vi "GetTerms3.vi"(0 "XRef":T11, 1 "State In":T9) -> (14 "Terms":T1)   [LabVIEW 2012, in "CRefScripting.lvlib" / "CRef Label Node.xnode"]
doc: "This ability VI is used to describe your terminals to LabVIEW. Terms is an array of clusters describing the XNode's terminals.\n ID: A unique string identifying the terminal.\n Name: The name of the terminal visible to the user. Remember to localize it.\n Type: The data type of the terminal (as a Variant). The data put in the variant will be used as the default for the input terminal if it's left unwired.\n Bounds: A rectangle defining the bounds of the terminal relative to the bounds of the XNode. The bounds must be within the bounds of the XNode, and for whiskers to draw properly, they must be flush with at least one side of the XNode.\n Input?: Indicates whether or not this terminals is an input.\n Required?: Indicates whether the user must wire this terminal for the XNode to not be broken. Ignored on outputs.\n Recommended?: Indicates whether the terminal is recommended.\n Hidden?: Indicates whether the terminal is hidden. When a terminal is hidden, it cannot be wired to via user interaction or scripting. However, if it is already wired to when the hidden flag is changed to true, it will remain wired.\n Adaptive?: Indicates that the term should change to match the type of its source if it is wired.\n Direction?: Indicates what direction the wire stub should point. Choose auto to let LV decide based on the terms bounds being on the nodes edge.\n \n The IDs are used by LabVIEW to keep track of your terminals. When you respecify your terminals, LabVIEW can tell whther terminals are new, deleted, or moved by the unique IDs. The order is irrelevant. If you move a terminal, then any wire connected to it will move with it.\n \n If you want to update your terminals, you should return the UpdateTerms reply in one of your ability VIs.\n\nDefault behavior: None.\n\nThis ability does not provide UI and OS messages are not handled."
uses:
  CRef Label Node.xnode
  <vilib>/XNodeSupport/XNodeXNodeRef.ctl
  State.ctl
  Core/Master Types.ctl
  <vilib>/XNodeSupport/XNodeTerm3Array.ctl
  <vilib>/XNodeSupport/XNodeTerm3.ctl
  <vilib>/XNodeSupport/XNodeString.ctl
  <vilib>/XNodeSupport/XNodeVariant.ctl
  <vilib>/XNodeSupport/XNodeRect32.ctl
  <vilib>/XNodeSupport/XNodeInt.ctl
  <vilib>/XNodeSupport/XNodeBool.ctl
  <vilib>/XNodeSupport/XNodeTermDirection.ctl
  <vilib>/XNodeSupport/NI_XNodeSupport.lvlib
  CRef.lvlib
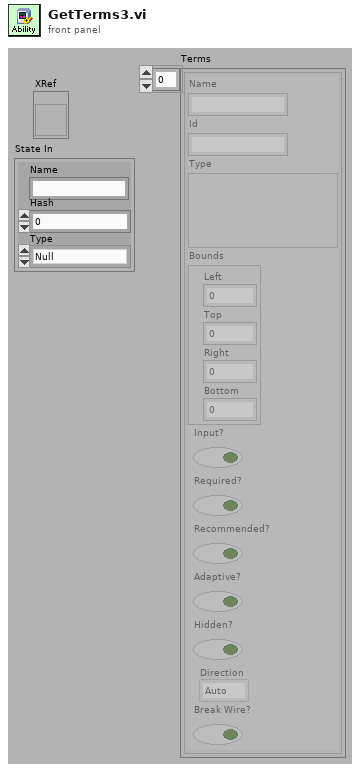
[diagram p1: front panel]
types:
  T1 = typedef "NI_XNodeSupport.lvlib/XNodeTerm3Array.ctl" = T2[]
  T2 = typedef "NI_XNodeSupport.lvlib/XNodeTerm3.ctl" = cluster{"Name":T3, "Id":T3, "Type":T4, "Bounds":T5, "Input?":T7, "Required?":T7, "Recommended?":T7, "Adaptive?":T7, "Hidden?":T7, "Direction":T8, "Break Wire?":T7}
  T3 = typedef "NI_XNodeSupport.lvlib/XNodeString.ctl" = string
  T4 = typedef "NI_XNodeSupport.lvlib/XNodeVariant.ctl" = variant
  T5 = typedef "NI_XNodeSupport.lvlib/XNodeRect32.ctl" = cluster{"Left":T6, "Top":T6, "Right":T6, "Bottom":T6}
  T6 = typedef "NI_XNodeSupport.lvlib/XNodeInt.ctl" = i32
  T7 = typedef "NI_XNodeSupport.lvlib/XNodeBool.ctl" = bool
  T8 = typedef "NI_XNodeSupport.lvlib/XNodeTermDirection.ctl" = enum32{"Auto", "Up", "Down", "Left", "Right", "Center"}
  T9 = typedef "CRefScripting.lvlib/CRef Label Node.xnode/State.ctl" = cluster{"Name":string, "Hash":u32, "Type":T10}
  T10 = typedef "CRef.lvlib/Master Types.ctl" = enum8{"Null", "Boolean", "U8", "I8", "U16", "I16", "U32", "I32", "U64", "I64", "Single", "Double", "Extended", "CSG", "CDB", "CXT", "Boolean(Def)", "U8(Def)", "I8(Def)", "U16(Def)", "I16(Def)", "U32(Def)", "I32(Def)", "Reserved Def", "Reserved Def1", "Single(Def)", "Double(Def)", "Reserved Def2", "Reserved Def3", "Reserved Def4", "Reserved Def5", "Unsigned(Def)", "Signed(Def)", "Real(Def)", "Reserved Def6", "Numeric(Def)", "String"}
  T11 = typedef "NI_XNodeSupport.lvlib/XNodeXNodeRef.ctl" = refnum<vi>
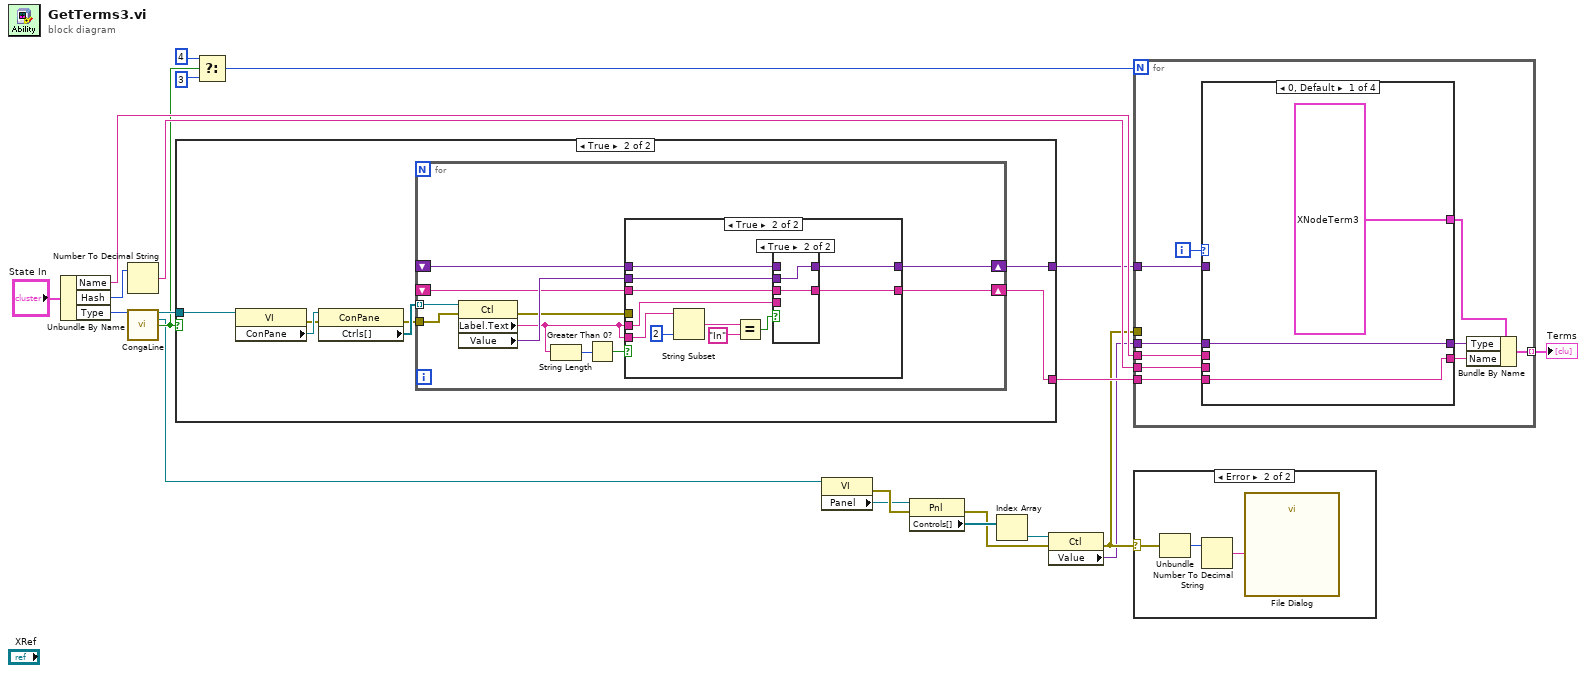
[diagram p0: block diagram]
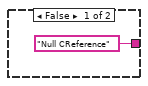
[diagram p3: hidden frame]
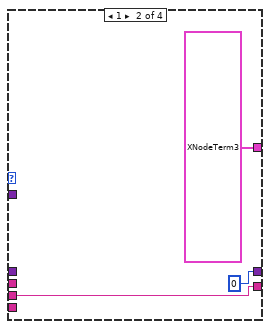
[diagram p6: hidden frame]
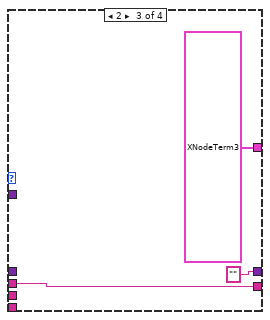
[diagram p7: hidden frame]
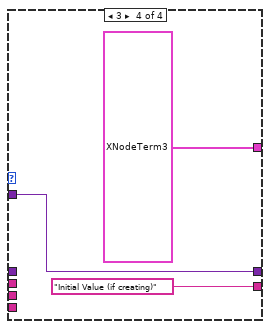
[diagram p8: hidden frame]
diagram:
  n1 = Unbundle By Name("State In") -> ("Name"=w18:string, "Hash"=w17:u32, "Type"=w20:T10)
  n2 = Number To Decimal String(number=w17) -> (decimal integer string=w16:string)  [unwired: 1 in]
  n3 = call "CongaLine.vi"("Type"=w20) -> ("vi reference"=w19:refnum<vi>, "CReference Ctl"=w8:refnum<vi>, "implemented?"=w9:bool)  [unwired: 11 in, 1 out]
  n4 = case shown="True" w9 {
    tunnel: w19 -> [_ w29]
    tunnel: [_ w26] -> w14
    tunnel: ["Null CReference" ("Label.ClassName") w25] -> w13
    frame False {
    }
    frame True {
      n5 = property class="VI"(reference=w29) -> (error out=w24:errorcluster, "ConPane"=w28:refnum<vi>)  [unwired: 1 in, 1 out]
      n6 = property class="ConPane"(reference=w28, error in=w24) -> (error out=w23:errorcluster, "Ctrls[]"=w27:refnum<vi>[])  [unwired: 1 out]
      n7 = for {
        tunnel: w27 -> [w40] mode=indexing
        shift-right: [w36] -> w26
        shift-left: _ -> [w35]
        shift-right: [w33] -> w25
        shift-left: _ -> [w32]
        tunnel: w23 -> [w31]
        n8 = property class="Ctl"(reference=w40, error in=w31) -> (error out=w30:errorcluster, "Label.Text"=w34:string, "Value"=w37:variant)  [unwired: 1 out]
        n9 = String Length(string=w34) -> (length=w39:i32)
        n10 = Greater Than 0?(x=w39) -> (x > 0?=w38:bool)
        n11 = case shown="True" w38 {
          tunnel: w37 -> [_ w48]
          tunnel: w34 -> [_ w52]
          tunnel: [w42 w47] -> w36
          tunnel: w35 -> [w42 w46]
          tunnel: w34 -> [_ w45]
          tunnel: [w41 w44] -> w33
          tunnel: w32 -> [w41 w43]
          tunnel: w30 -> [_ _]
          frame False {
          }
          frame True {
            n12 = String Subset(string=w52, length (rest)=2 ("length (rest)")) -> (substring=w51:string)  [unwired: 1 in]
            n13 = Equal?(x=w51, y="In") -> (x = y?=w49:bool)
            n14 = case shown="True" w49 {
              tunnel: w48 -> [_ w57]
              tunnel: [w55 w57] -> w47
              tunnel: w46 -> [w55 _]
              tunnel: [w54 w56] -> w44
              tunnel: w45 -> [w54 _]
              tunnel: w43 -> [_ w56]
              frame False {
              }
              frame True {
              }
            }
          }
        }
      }
    }
  }
  n15 = Select(t=4, s=w9, f=3) -> (s? t:f=w10:i32)
  n16 = property class="VI"(reference=w8) -> (error out=w7:errorcluster, "Panel"=w6:refnum<vi>)  [unwired: 1 in, 1 out]
  n17 = property class="Pnl"(reference=w6, error in=w7) -> (error out=w3:errorcluster, "Controls[]"=w5:refnum<vi>[])  [unwired: 1 out]
  n18 = Index Array(array=w5) -> (element=w4:refnum<vi>)  [unwired: 1 in]
  n19 = property class="Ctl"(reference=w4, error in=w3) -> (error out=w2:errorcluster, "Value"=w1:variant)  [unwired: 1 out]
  n20 = for {
    N: w10 -> [_]
    tunnel: [w64] -> w15 mode=indexing
    tunnel: w1 -> [w63]
    tunnel: w2 -> [_]
    tunnel: w14 -> [w62]
    tunnel: w13 -> [w61]
    tunnel: w18 -> [w59]
    tunnel: w16 -> [w58]
    i -> [w67]
    n21 = case shown="0, Default" w67 {
      tunnel: [w69 u32 0 "" w78] -> w65
      tunnel: [T2 {"Name"="", "Id"="CReference", "Type"=variant, "Bounds"={"Left"=18, "Top"=1, "Right"=31, "Bottom"=10}, "Input?"=FALSE, "Required?"=FALSE, "Recommended?"=FALSE, "Adaptive?"=FALSE, "Hidden?"=FALSE, "Direction"=enum."Right", "Break Wire?"=FALSE} ("Term 3") T2 {"Name"="", "Id"="Hash", "Type"=variant, "Bounds"={"Left"=21, "Top"=23, "Right"=31, "Bottom"=31}, "Input?"=FALSE, "Required?"=FALSE, "Recommended?"=FALSE, "Adaptive?"=FALSE, "Hidden?"=FALSE, "Direction"=enum."Right", "Break Wire?"=FALSE} ("Term 3") T2 {"Name"="", "Id"="Label", "Type"=variant, "Bounds"={"Left"=22, "Top"=11, "Right"=30, "Bottom"=20}, "Input?"=FALSE, "Required?"=FALSE, "Recommended?"=FALSE, "Adaptive?"=FALSE, "Hidden?"=FALSE, "Direction"=enum."Right", "Break Wire?"=FALSE} ("Term 3") T2 {"Name"="", "Id"="Initial Value", "Type"=variant, "Bounds"={"Left"=6, "Top"=11, "Right"=16, "Bottom"=22}, "Input?"=TRUE, "Required?"=FALSE, "Recommended?"=TRUE, "Adaptive?"=FALSE, "Hidden?"=FALSE, "Direction"=enum."Left", "Break Wire?"=FALSE} ("Term 3")] -> w66
      tunnel: w63 -> [w69 _ _ _]
      tunnel: w62 -> [_ _ _ w78]
      tunnel: w61 -> [w68 _ _ _]
      tunnel: [w68 w71 w74 "Initial Value (if creating)" ("Name")] -> w60
      tunnel: w59 -> [_ _ w74 _]
      tunnel: w58 -> [_ w71 _ _]
      frame 0, Default {
      }
      frame 1 {
      }
      frame 2 {
      }
      frame 3 {
      }
    }
    n22 = Bundle By Name(cluster=w66, "Type"=w65, "Name"=w60) -> (w64:T2)
  }
  "Terms" <- w15
  n23 = case shown="Error" w2 {
    selector: w2 -> [_ w82]
    frame No Error {
    }
    frame Error {
      n24 = Unbundle(w82) -> ("code"=w81:i32)  [unwired: 2 out]
      n25 = Number To Decimal String(number=w81) -> (decimal integer string=w80:string)  [unwired: 1 in]
      n26 = call "File Dialog"("prompt"=w80) -> ()  [unwired: 11 in, 4 out]
    }
  }
